vi "Get Last Error.vi"(8 "error in (no error)":errorcluster, 11 "Nominal Streaming in":refnum<class "Stream.lvclass">) -> (0 "error out":errorcluster, 3 "Nominal Streaming out":refnum<class "Stream.lvclass">)   [LabVIEW 2020, in "Nominal Streaming.lvlib" / "Stream.lvclass"]
uses:
  Stream.lvclass
  Stream.lvclass/Stream.ctl
  bin/lib_nominal-streaming-lv_64.dll
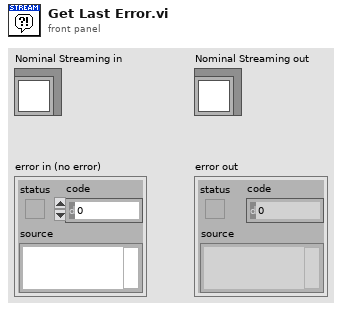
[diagram p1: front panel]
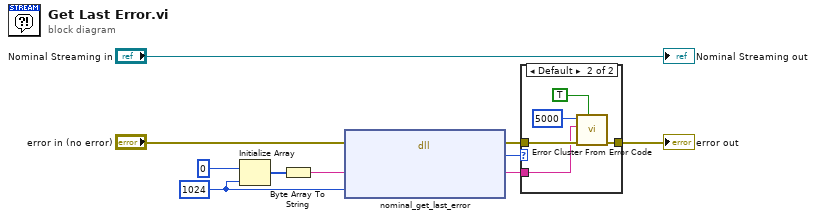
[diagram p0: block diagram]
diagram:
  w9 = u64 1024 ("buffer_size")
  n1 = Initialize Array(u8 0, w9) -> (w8:u8[])
  n2 = Byte Array To String(unsigned byte array=w8) -> (string=w7:string)
  n3 = dll-call lib="C:/code/nominal-streaming-labview-ffi/lv_src/bin/lib_nominal-streaming-lv_*.*" fn="nominal_get_last_error"(error in="error in (no error)", "buffer"=w7, "buffer_size"=w9) -> (error out=w5:errorcluster, "return type"=w2:i32, "buffer"=w3:string)  [unwired: 3 in, 1 out]
  n4 = case shown="Default" w2 {
    tunnel: w5 -> [w11 w16]
    tunnel: [w11 w15] -> w4
    tunnel: w3 -> [_ w14]
    frame -1 {
    }
    frame Default {
      n5 = call <vilib>:"Error Cluster From Error Code.vi"("show call chain? (False)"=TRUE, "error in (no error)"=w16, "error message (\"\")"=w14, "error code (0)"=5000) -> ("error out"=w15:errorcluster)  [unwired: 5 in]
    }
  }
  "error out" <- w4
  "Nominal Streaming out" <- "Nominal Streaming in"
